vi "Loading Loop.vi"(7 "ctrl index":i32, 10 "Q":refnum<queue>, 11 "owner VI":refnum<vi>) -> ()   [LabVIEW 2017]
uses:
  Controls/Error Codes List Window States.ctl
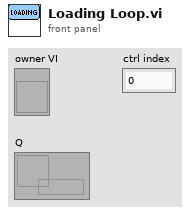
[diagram p1: front panel]
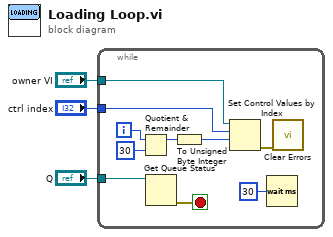
[diagram p0: block diagram]
diagram:
  n1 = while {
    tunnel: "Q" -> [w10]
    tunnel: "ctrl index" -> [w8]
    tunnel: "owner VI" -> [w6]
    i -> [w13]
    stop <- w5 stop-if-true
    n2 = Quotient & Remainder(x=w13, y=30) -> (x-y*floor(x/y)=w11:i32)  [unwired: 1 out]
    n3 = Get Queue Status(queue=w10) -> (error out=w5:errorcluster)  [unwired: 2 in, 7 out]
    n4 = To Unsigned Byte Integer(number=w11) -> (unsigned 8bit integer=w9:u8)
    n5 = Set Control Values by Index(0:w6, 1:w8, 2:w9) -> (11:w7:errorcluster)  [unwired: 1 in]
    n6 = Wait (ms)(milliseconds to wait=u32 30) -> ()  [unwired: 1 out]
    n7 = call <vilib>:"Clear Errors.vi"("error in (no error)"=w7) -> ()  [unwired: 5 in, 2 out]
  }
